vi "initialize.vi"(0 "HGF_ImaqUsb":refnum<class "HGF_ImaqUsb.lvclass">, 3 "initializationData":variant, 5 "error in (no error)":errorcluster, 7 "binaryString":string, 8 "I8 Array":i8[](array[numeric]), 9 "prependSize? (T)":bool, 11 "byteOrder (0:big-endian, network order)":T1(ring)) -> (14 "dup HGF_ImaqUsb":refnum<class "HGF_ImaqUsb.lvclass">, 17 "found?":bool, 19 "error out":errorcluster)   [LabVIEW 2009, in "HGF_ImaqUsb.lvclass"]
doc: "This is a dynamic dispatch VI to be implemented by child classes to initialize their attributes.\n\n<B>Recommendation:</B> Use Variant for initialization data."
uses:
  HGF_ImaqUsb.lvclass
  HGF_IMAQDevice/HGF_IMAQDevice.lvclass
  HGF_ImaqUsb.lvclass/HGF_ImaqUsb.ctl
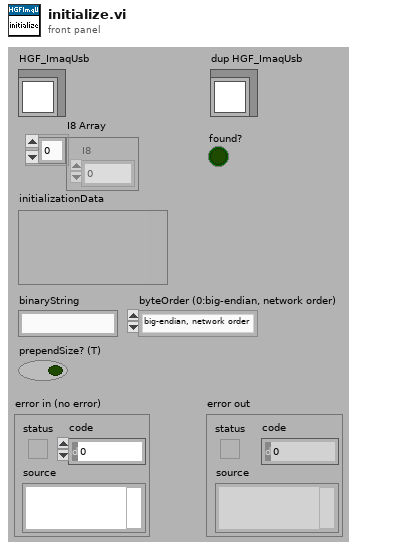
[diagram p1: front panel]
types:
  T1 = enum16{"big-endian, network order", "native, host order", "little-endian"}
  T2 = typedef "IMAQ USB.ctl" = refnum<k1>
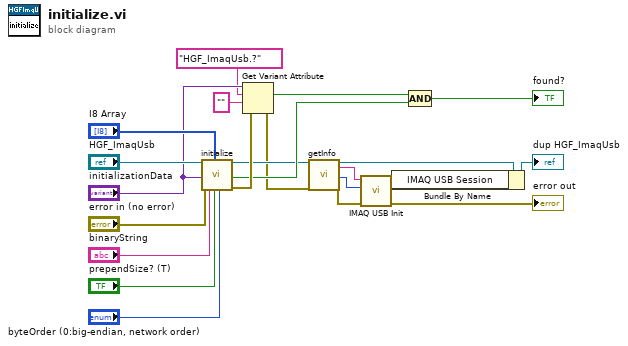
[diagram p0: block diagram]
diagram:
  n1 = call-parent "initialize.vi"("HGF_IMAQDevice"="HGF_ImaqUsb", "initializationData"="initializationData", "error in (no error)"="error in (no error)", "binaryString"="binaryString", "I8 Array"="I8 Array", "prependSize? (T)"="prependSize? (T)", "byteOrder (0:big-endian, network order)"="byteOrder (0:big-endian, network order)") -> ("dup HGF_IMAQDevice"=w8:refnum<class "HGF_ImaqUsb.lvclass">, "found?"=w13:bool, "error out"=w15:errorcluster)  [unwired: 10 out]
  n2 = Get Variant Attribute(Variant="initializationData", name="HGF_ImaqUsb.?", default value (empty Variant)="", error in=w15) -> (found=w14:bool, error out=w6:errorcluster)  [unwired: 2 out]
  n3 = call "getInfo.vi"("HGF_IMAQDevice"=w8, "error in (no error)"=w6) -> ("dup HGF_IMAQDevice"=w7:refnum<class "HGF_ImaqUsb.lvclass">, "cameraName"=w5:string, "videoMode"=w2:i32, "error out"=w4:errorcluster)  [unwired: 12 in, 2 out]
  n4 = call <vilib>:"IMAQ USB Init.vi"("error in (no error)"=w4, "Video Mode"=w2, "USB Camera Name"=w5) -> ("error out"=→"error out":errorcluster, "IMAQ USB Session Out"=w1:T2)  [unwired: 7 out]
  n5 = Bundle By Name(cluster=w7, "IMAQ USB Session"=w1) -> (→"dup HGF_ImaqUsb":refnum<class "HGF_ImaqUsb.lvclass">)
  n6 = Compound Arithmetic op=AND(w14, w13) -> (→"found?":bool)
